vi "_PC_Pub_GenerateTimeRandom.vi"() -> (0 "hex integer string":string)   [LabVIEW 2018]
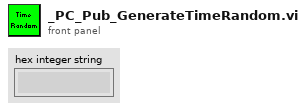
[diagram p1: front panel]
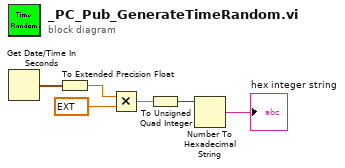
[diagram p0: block diagram]
diagram:
  n1 = Get Date/Time In Seconds() -> (seconds since 1Jan1904=w6:timestamp)
  n2 = To Extended Precision Float(1:w6) -> (0:w5:ext)
  n3 = Multiply(x=w5, y=ext 1000.0) -> (x*y=w3:ext)
  n4 = To Unsigned Quad Integer(1:w3) -> (0:w2:u64)
  n5 = Number To Hexadecimal String(2:w2) -> (0:→"hex integer string":string)  [unwired: 1 in]
